vi "Extract Command Type.vi"(8 "error in (no error)":errorcluster, 11 "Command field in":string) -> (0 "error out":errorcluster, 1 "Command valid?":bool, 2 "Command Type":T2=enum."instrument_control", 3 "Command":T1, 5 "command received":string)   [LabVIEW 2019, in "mmW_commands.lvlib"]
uses:
  mmW_commands.lvlib
  TypeDefs/commands.ctl
  TypeDefs/_depr_commands_environment_control.ctl
  TypeDefs/command_types.ctl
  <vilib>/Field R&D Services/Logger/Field_RnD_Services_Logger_Toolkit.lvlib
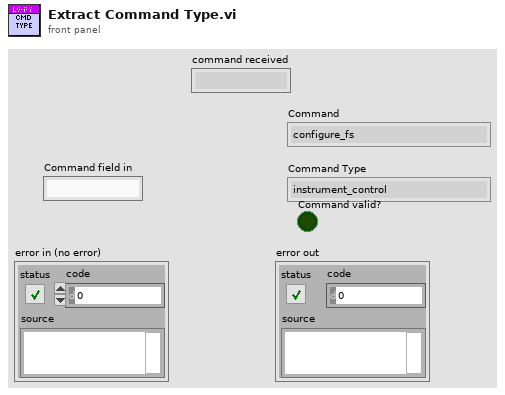
[diagram p1: front panel]
types:
  T1 = typedef "mmW_commands.lvlib/commands.ctl" = enum16{"configure_fs", "configure_rf", "configure_trigger", "equalization_enable", "equalization_start", "lo_sync_enable", "equalization_stop", "get_instrument_status", "get_versions", "initialize_hw", "pop_rx", "set_log_level", "Shutdown", "start", "start_instrument_app", "stop", "transceive", "trigger_burst", "trigger_sync_enable", "Write TX", "resp_generic", "resp_waveform"}
  T2 = typedef "mmW_commands.lvlib/command_types.ctl" = enum16{"invalid_command", "instrument_control", "environment_control", "response"}
  T3 = typedef "mmW_commands.lvlib/_depr_commands_environment_control.ctl" = enum16{"get_instrument_status", "get_versions", "start_instrument_app"}
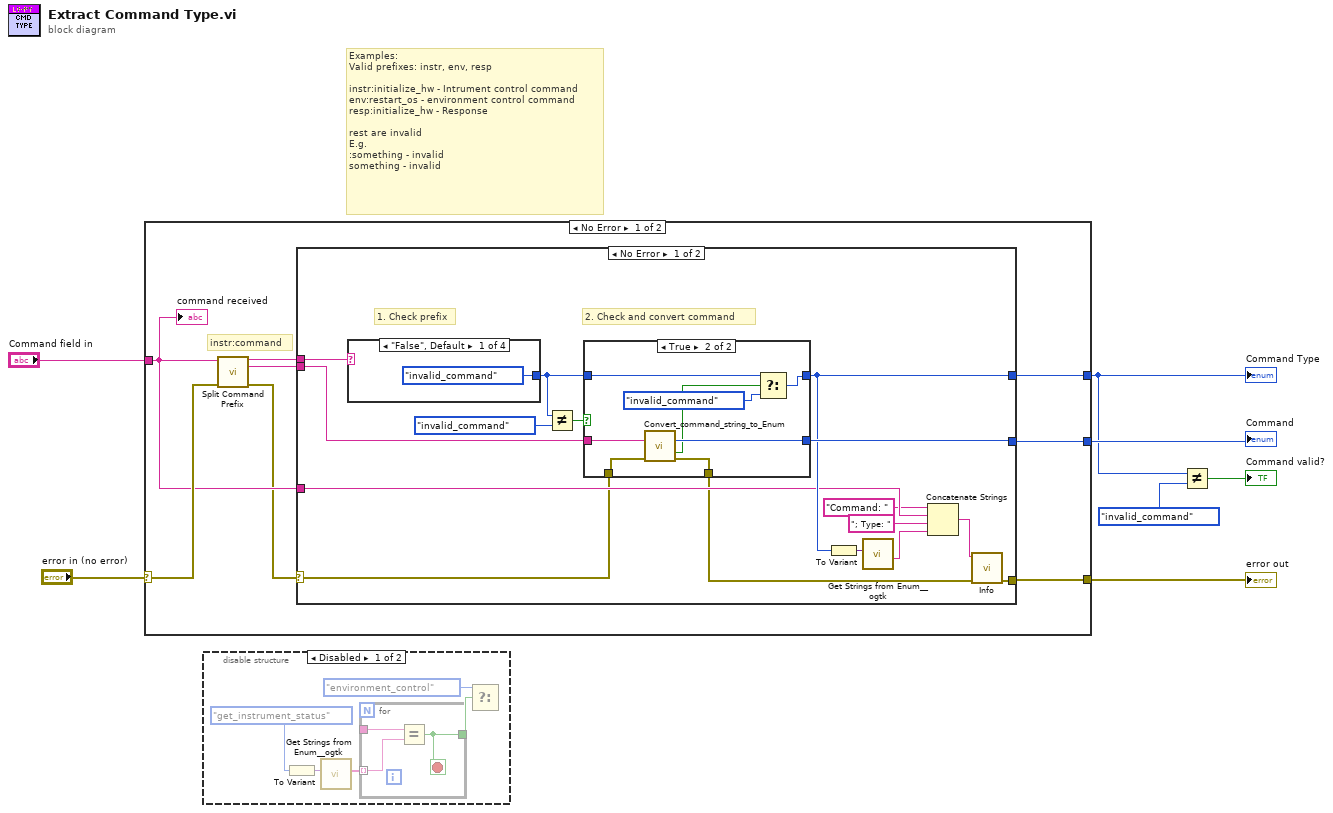
[diagram p0: block diagram]
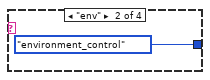
[diagram p4: hidden frame]
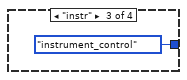
[diagram p5: hidden frame]
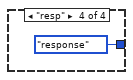
[diagram p6: hidden frame]
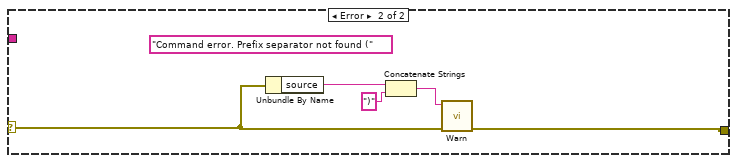
[diagram p7: hidden frame]
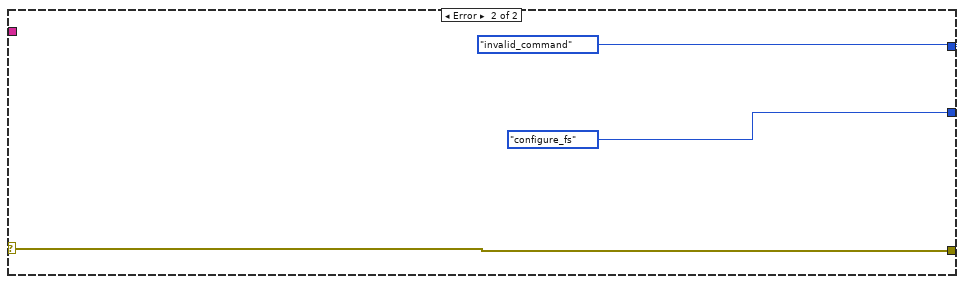
[diagram p8: hidden frame]
diagram:
  # "Examples:\nValid prefixes: instr, env, resp\n\ninstr:initialize_hw - Intrument control command\nenv:restart_os - environment control command\nresp:initialize_hw - Response\n\nrest are invalid\nE.g.\n:something - invalid\nsomething - invalid"
  n1 = case shown="No Error" "error in (no error)" {
    selector: "error in (no error)" -> [w12 w53]
    tunnel: [w13 w53] -> w7
    tunnel: [w14 command_types."invalid_command" ("Command_Types")] -> w3
    tunnel: "Command field in" -> [w11 _]
    tunnel: [w15 commands."configure_fs" ("mmW_instrument_commands")] -> w4
    frame No Error {
      # "instr:command"
      n2 = call "Split Command Prefix.vi"("command string in"=w11, "error in"=w12) -> ("command prefix"=w9:string, "command out"=w8:string, "error out"=w10:errorcluster)  [unwired: 11 in]
      n3 = case shown="No Error" w10 {
        selector: w10 -> [w16 w47]
        tunnel: [w31 _] -> w15
        tunnel: w9 -> [w30 _]
        tunnel: w8 -> [w29 _]
        tunnel: [w28 _] -> w14
        tunnel: [w27 w46] -> w13
        tunnel: w11 -> [w26 _]
        frame No Error {
          # "2. Check and convert command"
          # "1. Check prefix"
          n4 = case shown="\"False\", Default" w30 {
            tunnel: [command_types."invalid_command" ("s? t:f") command_types."environment_control" ("s? t:f") command_types."instrument_control" ("s? t:f") command_types."response" ("s? t:f")] -> w24
            frame "False", Default {
            }
            frame "env" {
            }
            frame "instr" {
            }
            frame "resp" {
            }
          }
          n5 = Not Equal?(x=w24, y=command_types."invalid_command") -> (x != y?=w23:bool)
          n6 = case shown="True" w23 {
            tunnel: w16 -> [w32 w41]
            tunnel: [w32 w40] -> w17
            tunnel: [_ w39] -> w31
            tunnel: w29 -> [_ w34]
            tunnel: w24 -> [w33 w37]
            tunnel: [w33 w35] -> w28
            frame False {
            }
            frame True {
              n7 = call "Convert_command_string_to_Enum.vi"("Command field in"=w34, "error in (no error)"=w41) -> ("mmW_instrument_commands"=w39:T1, "Found in Enum?"=w38:bool, "error out"=w40:errorcluster)  [unwired: 11 in]
              n8 = Select(t=w37, s=w38, f=command_types."invalid_command" ("y")) -> (s? t:f=w35:T2)
            }
          }
          n9 = To Variant(anything=w28) -> (Variant=w21:variant)
          n10 = call <userlib>:"Get Strings from Enum__ogtk.vi"("Enum"=w21) -> ("String Value"=w20:string)  [unwired: 7 in, 3 out]
          n11 = Concatenate Strings("Command: " ("string"), w26, "; Type: " ("string"), w20) -> (w22:string)
          n12 = call <vilib>:"Info.vi"("Error In"=w17, "Message"=w22) -> ("Error Out"=w27:errorcluster)  [unwired: 9 in]
        }
        frame Error {
          (unwired) "Command error. Prefix separator not found ("
          n13 = Unbundle By Name(w47) -> ("source"=w48:string)
          n14 = Concatenate Strings(w48, ")" ("string")) -> (w49:string)
          n15 = call <vilib>:"Warn.vi"("Error In"=w47, "Message"=w49) -> ("Error Out"=w46:errorcluster)  [unwired: 9 in]
        }
      }
      "command received" <- w11
    }
    frame Error {
    }
  }
  "error out" <- w7
  "Command Type" <- w3
  "Command" <- w4
  n16 = disable-structure shown="Disabled" {
    frame Disabled {
      n17 = To Variant(anything=_depr_commands_environment_control."get_instrument_status" ("Environment_control_commands")) -> (Variant=w57:variant)
      n18 = call <userlib>:"Get Strings from Enum__ogtk.vi"("Enum"=w57) -> ("Enum Strings"=w58:string[])  [unwired: 7 in, 3 out]
      n19 = for {
        tunnel: _ -> [w61]
        tunnel: w58 -> [w60] mode=indexing
        tunnel: [w59] -> w55
        stop <- w59 stop-if-true
        n20 = Equal?(x=w61, y=w60) -> (x = y?=w59:bool)
      }
      n21 = Select(t=command_types."environment_control" ("Command_Types"), s=w55) -> ()  [unwired: 1 in, 1 out]
    }
    frame Enabled {
    }
  }
  n22 = Not Equal?(x=w3, y=command_types."invalid_command") -> (x != y?=→"Command valid?":bool)
